vi "DAC return end times.vi"(1 "Text DAC Array In":T1(array[cluster])=[{"start voltage (V)"="", "start time (ms)"="", "Enable DAC"=FALSE, "Hinge points"=[]}, {"start voltage (V)"="", "start time (ms)"="", "Enable DAC"=TRUE, "Hinge points"=[]}, {"start voltage (V)"="", "start time (ms)"="", "Enable DAC"=TRUE, "Hinge points"=[]}, {"start voltage (V)"="", "start time (ms)"="", "Enable DAC"=TRUE, "Hinge points"=[]}, {"start voltage (V)"="", "start time (ms)"="", "Enable DAC"=FALSE, "Hinge points"=[]}, {"start voltage (V)"="", "start time (ms)"="", "Enable DAC"=TRUE, "Hinge points"=[]}, {"start voltage (V)"="", "start time (ms)"="", "Enable DAC"=TRUE, "Hinge points"=[]}, {"start voltage (V)"="", "start time (ms)"="", "Enable DAC"=FALSE, "Hinge points"=[]}] caption="text DAC Array In" {"Hinge points"."transition" items=["Step", "Ramp", "Exp"]}, 2 "number DAC Array In":T2(array[cluster])) -> (0 "Text DAC Array Out":T1(array[cluster])=[{"start voltage (V)"="", "start time (ms)"="", "Enable DAC"=FALSE, "Hinge points"=[]}, {"start voltage (V)"="", "start time (ms)"="", "Enable DAC"=TRUE, "Hinge points"=[]}, {"start voltage (V)"="", "start time (ms)"="", "Enable DAC"=TRUE, "Hinge points"=[]}, {"start voltage (V)"="", "start time (ms)"="", "Enable DAC"=TRUE, "Hinge points"=[]}, {"start voltage (V)"="", "start time (ms)"="", "Enable DAC"=FALSE, "Hinge points"=[]}, {"start voltage (V)"="", "start time (ms)"="", "Enable DAC"=TRUE, "Hinge points"=[]}, {"start voltage (V)"="", "start time (ms)"="", "Enable DAC"=TRUE, "Hinge points"=[]}, {"start voltage (V)"="", "start time (ms)"="", "Enable DAC"=FALSE, "Hinge points"=[]}] {"Hinge points"."transition" items=["Step", "Ramp", "Exp"]})   [LabVIEW 2010]
doc: "Takes the end times from a DAC array with numbers and puts them into a DAC array with text. Inputs are the DAC array with numbers (obtained from AO array which calculates end times) and the DAC array with text. Output is the new DAC array with text."
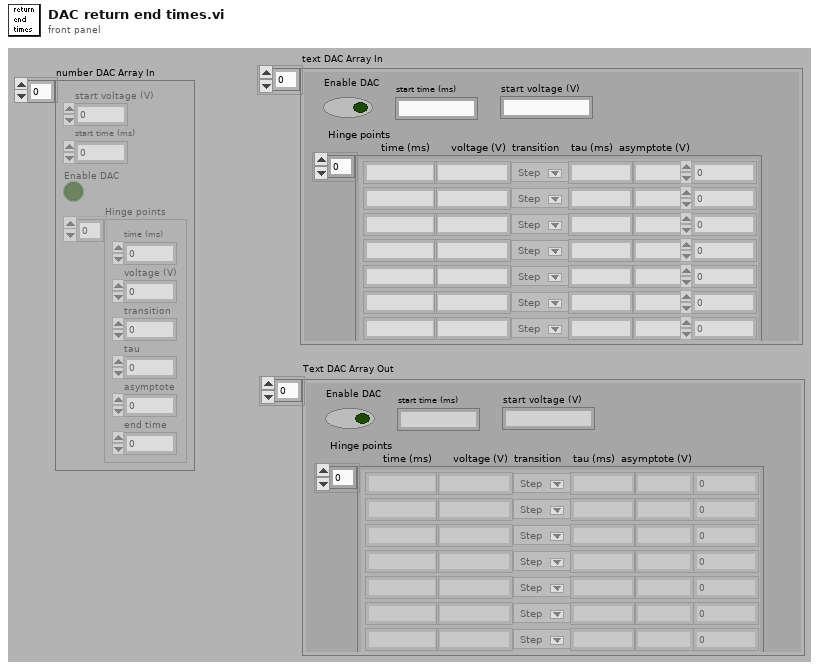
[diagram p1: front panel]
types:
  T1 = cluster{"start voltage (V)":string, "start time (ms)":string, "Enable DAC":bool, "Hinge points":cluster{"time (ms)":string, "voltage (V)":string, "transition":u16, "tau":string, "asymptote":string, "end time":dbl}[]}[]
  T2 = cluster{"start voltage (V)":dbl, "start time (ms)":dbl, "Enable DAC":bool, "Hinge points":cluster{"time (ms)":dbl, "voltage (V)":dbl, "transition":u16, "tau":dbl, "asymptote":dbl, "end time":dbl}[]}[]
  T3 = cluster{"time (ms)":string, "voltage (V)":string, "transition":u16, "tau":string, "asymptote":string, "end time":dbl}[]
  T4 = cluster{"time (ms)":dbl, "voltage (V)":dbl, "transition":u16, "tau":dbl, "asymptote":dbl, "end time":dbl}[]
  T5 = cluster{"time (ms)":string, "voltage (V)":string, "transition":u16, "tau":string, "asymptote":string, "end time":dbl}
  T6 = cluster{"start voltage (V)":string, "start time (ms)":string, "Enable DAC":bool, "Hinge points":cluster{"time (ms)":string, "voltage (V)":string, "transition":u16, "tau":string, "asymptote":string, "end time":dbl}[]}
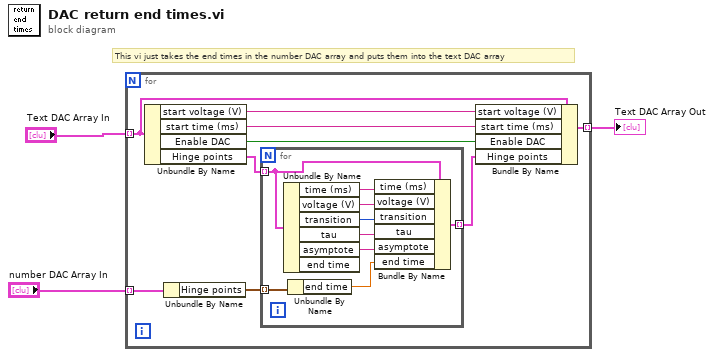
[diagram p0: block diagram]
diagram:
  # "This vi just takes the end times in the number DAC array and puts them into the text DAC array"
  n1 = for {
    tunnel: "number DAC Array In" -> [w12] mode=indexing
    tunnel: "Text DAC Array In" -> [w10] mode=indexing
    tunnel: [w4] -> w1 mode=indexing
    n2 = Unbundle By Name(w10) -> ("start voltage (V)"=w9:string, "start time (ms)"=w8:string, "Enable DAC"=w7:bool, "Hinge points"=w6:T3)
    n3 = Unbundle By Name(w12) -> ("Hinge points"=w11:T4)
    n4 = for {
      tunnel: w11 -> [w21] mode=indexing
      tunnel: w6 -> [w20] mode=indexing
      tunnel: [w13] -> w5 mode=indexing
      n5 = Unbundle By Name(w20) -> ("time (ms)"=w19:string, "voltage (V)"=w18:string, "transition"=w17:u16, "tau"=w16:string, "asymptote"=w15:string)  [unwired: 1 out]
      n6 = Unbundle By Name(w21) -> ("end time"=w14:dbl)
      n7 = Bundle By Name(cluster=w20, "time (ms)"=w19, "voltage (V)"=w18, "transition"=w17, "tau"=w16, "asymptote"=w15, "end time"=w14) -> (w13:T5)
    }
    n8 = Bundle By Name(cluster=w10, "start voltage (V)"=w9, "start time (ms)"=w8, "Enable DAC"=w7, "Hinge points"=w5) -> (w4:T6)
  }
  "Text DAC Array Out" <- w1
